vi "WFStringToInt.vi"(10 "WaveFormType":string) -> (2 "WaveFormTypeInt":u16)   [LabVIEW 2010]
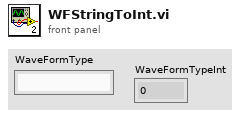
[diagram p1: front panel]
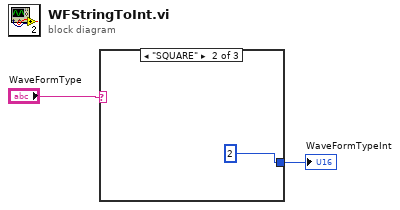
[diagram p0: block diagram]
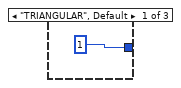
[diagram p2: hidden frame]
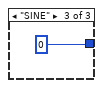
[diagram p3: hidden frame]
diagram:
  n1 = case shown="\"SQUARE\"" "WaveFormType" {
    tunnel: [1 2 0] -> w1
    frame "TRIANGULAR", Default {
    }
    frame "SQUARE" {
    }
    frame "SINE" {
    }
  }
  "WaveFormTypeInt" <- w1
